vi "Read Datagram.vi"(8 "error in (no error)":errorcluster, 11 "mqttCmd in":refnum<class "BaseMqttMsg.lvclass">) -> (0 "error out":errorcluster, 2 "Datagram":u8[](array[numeric]) format="%x", 3 "mqttCmd out":refnum<class "BaseMqttMsg.lvclass">)   [LabVIEW 2020]
uses:
  BaseMqttMsg.lvclass
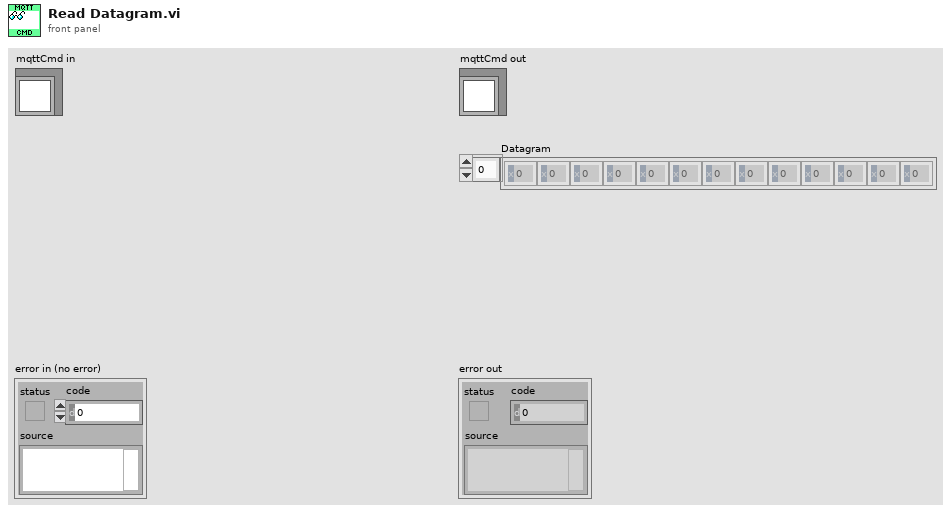
[diagram p1: front panel]
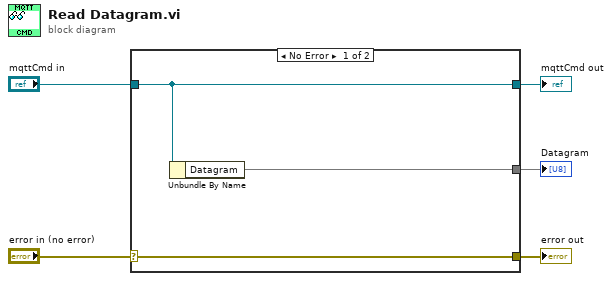
[diagram p0: block diagram]
diagram:
  n1 = case shown="No Error" "error in (no error)" {
    selector: "error in (no error)" -> [w8 w9]
    tunnel: [w8 w9] -> w4
    tunnel: [w7 w10] -> w2
    tunnel: "mqttCmd in" -> [w7 w10]
    tunnel: [w6 _] -> w1
    frame No Error {
      n2 = Unbundle By Name(w7) -> ("Datagram"=w6)
    }
    frame Error {
    }
  }
  "error out" <- w4
  "mqttCmd out" <- w2
  "Datagram" <- w1
